vi "auto avance recule.vi"(8 "temps de changement de direction":dbl, 9 "temps":dbl, 10 "vitesse gauche":dbl, 11 "vitesse droit":dbl) -> ()   [LabVIEW 2015]
uses:
  <vilib>/Rock Robotics/WPI/Utilities/WPI_GetSetVariantRefNum.vi
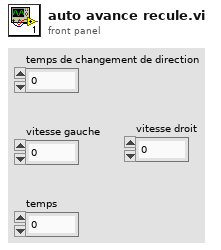
[diagram p1: front panel]
types:
  T1 = typedef "WPI_RobotDriveDevRef.ctl" = cluster{"DevStatus":errorcluster, "Motors[]":T2[], "Square Inputs":bool, "Max Output":dbl}
  T2 = typedef "WPI_MotorControlDeviceRef.ctl" = cluster{"DeviceStatus":errorcluster, "Type":T3, "PWM":cluster{"PWM Channel":T4, "DeadBand":T5}, "CAN":cluster{"Device Number":u8, "Control Mode":T6, "Semaphore":T7, "Max Vout":dbl, "TalonSRX Control Mode":T8}, "Invert":bool}
  T3 = typedef "WPI_MotorControlType.ctl" = enum16{"PWM", "CAN", "CANTalonSRX"}
  T4 = typedef "FPGA_DIOPWMChannel.ctl" = enum8{"PWM 0", "PWM 1", "PWM 2", "PWM 3", "PWM 4", "PWM 5", "PWM 6", "PWM 7", "PWM 8", "PWM 9", "PWM MXP 0", "PWM MXP 1", "PWM MXP 2", "PWM MXP 3", "PWM MXP 4", "PWM MXP 5", "PWM MXP 6", "PWM MXP 7", "PWM MXP 8", "PWM MXP 9", "Invalid"}
  T5 = typedef "WPI_PWMDeadband.ctl" = cluster{"Name":string, "maxPositivePwm":i32, "minPositivePwm":i32, "centerPwm":i32, "maxNegativePwm":i32, "minNegativePwm":i32, "angularRange":u16}
  T6 = typedef "WPI_CANJaguar_ControlMode.ctl" = enum8{"Percent VBus", "Current", "Speed", "Position", "Voltage"}
  T7 = typedef "Semaphore RefNum" = refnum<k1>
  T8 = typedef "WPI_CANTalonSRX_APIControlMode.ctl" = enum8{"Percent VBus", "Speed", "Position", "Slave", "Unchanged / Invalid", "Voltage Compensation", "Current", "Motion Profile"}
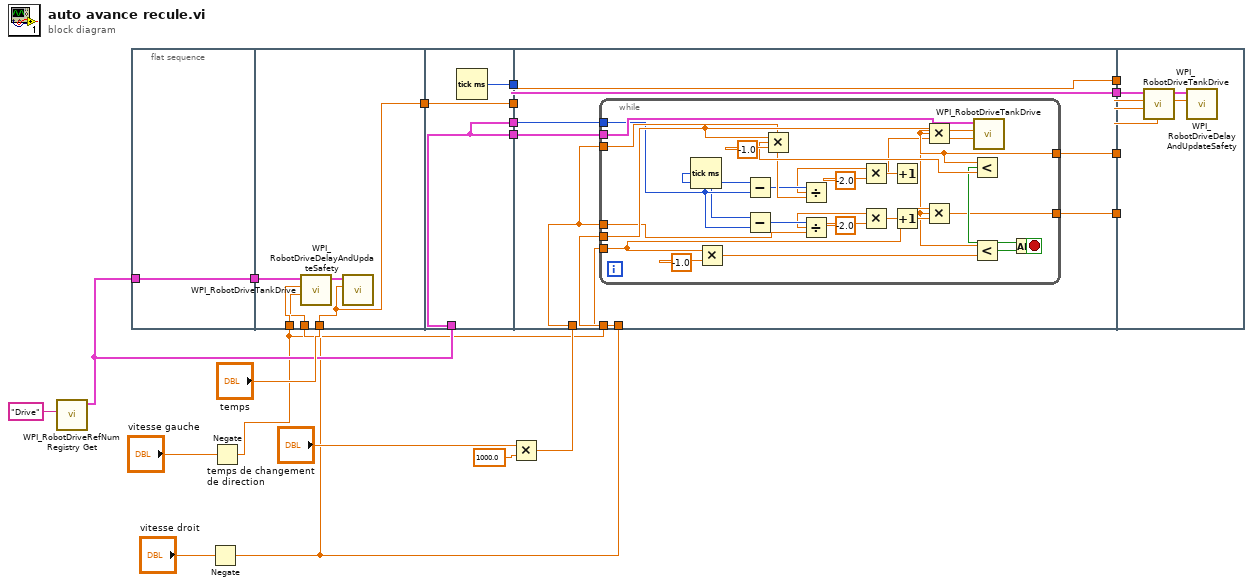
[diagram p0: block diagram]
diagram:
  n1 = call <vilib>:"WPI_RobotDriveRefNum Registry Get.vi"("refnum name"="Drive") -> ("RobotDriveDevRef"=w9:T1)  [unwired: 9 in, 1 out]
  n2 = flat-sequence {
    tunnel: w9 -> [w21]
    tunnel: [w21] -> w20
    tunnel: w20 -> [w25]
    tunnel: w2 -> [w24]
    tunnel: [w23] -> w19
    tunnel: "temps" -> [w23]
    tunnel: w3 -> [w22]
    tunnel: [w29] -> w18
    tunnel: [w28] -> w17
    tunnel: w9 -> [w28]
    tunnel: [w28] -> w16
    tunnel: w19 -> [w27]
    tunnel: [w27] -> w15
    tunnel: w18 -> [w38]
    tunnel: w17 -> [w37]
    tunnel: w16 -> [w36]
    tunnel: [w36] -> w14
    tunnel: w2 -> [w35]
    tunnel: [w34] -> w13
    tunnel: w15 -> [w33]
    tunnel: [w33] -> w12
    tunnel: w6 -> [w32]
    tunnel: w3 -> [w31]
    tunnel: [w30] -> w5
    tunnel: w14 -> [w68]
    tunnel: w13 -> [w67]
    tunnel: w12 -> [w66]
    tunnel: w5 -> [w65]
    frame #0 {
    }
    frame #1 {
      n3 = call <vilib>:"WPI_RobotDriveTankDrive.vi"("Right axis value"=w22, "Left axis value"=w24, "RobotDriveDevRef"=w25) -> ("RobotDriveDevRef"=w26:T1)  [unwired: 6 in, 2 out]
      n4 = call <vilib>:"WPI_RobotDriveDelayAndUpdateSafety.vi"("Delay (s)"=w23, "RobotDriveDevRef"=w26) -> ()  [unwired: 8 in, 2 out]
    }
    frame #2 {
      n5 = Tick Count (ms)() -> (millisecond timer value=w29:u32)
    }
    frame #3 {
      n6 = while {
        tunnel: w38 -> [w43]
        tunnel: w37 -> [w44]
        tunnel: w35 -> [w63]
        tunnel: [w61] -> w34
        tunnel: w32 -> [w60]
        tunnel: w32 -> [w42]
        tunnel: w31 -> [w41]
        tunnel: [w40] -> w30
        stop <- w47 stop-if-true
        n7 = Tick Count (ms)() -> (millisecond timer value=w39:u32)
        n8 = Multiply(x=w41, y=-1.0) -> (x*y=w53:dbl)
        n9 = Subtract(x=w39, y=w43) -> (x-y=w59:u32)
        n10 = Subtract(x=w39, y=w43) -> (x-y=w52:u32)
        n11 = Multiply(x=w63, y=-1.0) -> (x*y=w62:dbl)
        n12 = Divide(x=w59, y=w60) -> (x/y=w57:dbl)
        n13 = Divide(x=w52, y=w42) -> (x/y=w50:dbl)
        n14 = Multiply(x=w57, y=-2.0) -> (x*y=w56:dbl)
        n15 = Multiply(x=w50, y=-2.0) -> (x*y=w49:dbl)
        n16 = Increment(x=w56) -> (x+1=w55:dbl)
        n17 = Increment(x=w49) -> (x+1=w48:dbl)
        n18 = Multiply(x=w63, y=w55) -> (x*y=w61:dbl)
        n19 = Multiply(x=w41, y=w48) -> (x*y=w40:dbl)
        n20 = Less?(x=w61, y=w62) -> (x < y?=w46:bool)
        n21 = Less?(x=w40, y=w53) -> (x < y?=w45:bool)
        n22 = call <vilib>:"WPI_RobotDriveTankDrive.vi"("Right axis value"=w40, "Left axis value"=w61, "RobotDriveDevRef"=w44) -> ()  [unwired: 6 in, 3 out]
        n23 = And(x=w46, y=w45) -> (x .and. y?=w47:bool)
      }
    }
    frame #4 {
      n24 = call <vilib>:"WPI_RobotDriveTankDrive.vi"("Right axis value"=w65, "Left axis value"=w67, "RobotDriveDevRef"=w68) -> ("RobotDriveDevRef"=w69:T1)  [unwired: 6 in, 2 out]
      n25 = call <vilib>:"WPI_RobotDriveDelayAndUpdateSafety.vi"("Delay (s)"=w66, "RobotDriveDevRef"=w69) -> ()  [unwired: 8 in, 2 out]
    }
  }
  n26 = Negate(x="vitesse droit") -> (-x=w3:dbl)
  n27 = Negate(x="vitesse gauche") -> (-x=w2:dbl)
  n28 = Multiply(x="temps de changement de direction", y=1000.0) -> (x*y=w6:dbl)
